vi "Tone (G3)-Create.vi"(0 "Tone Class in":T1, 5 "Sampling Rate (Hz)":dbl, 7 "Npts":i32, 9 "RepNum":i32, 11 "error in (no error)":errorcluster) -> (4 "Tone Class out":T1, 6 "Waveform":dbl[](array[numeric]), 15 "error out":errorcluster)   [LabVIEW 2020]
uses:
  Tone.Properties.ctl
  <vilib>/Analysis/NI_AALBase.lvlib
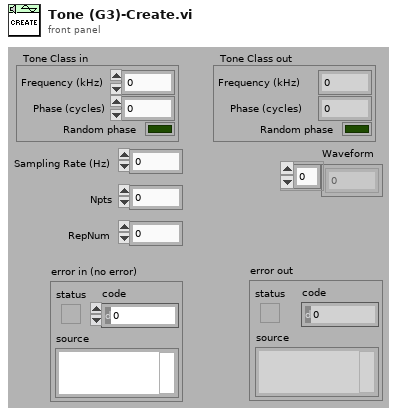
[diagram p1: front panel]
types:
  T1 = typedef "Tone.Properties.ctl" = cluster{"Frequency (kHz)":dbl, "Phase (cycles)":dbl, "Random phase":bool}
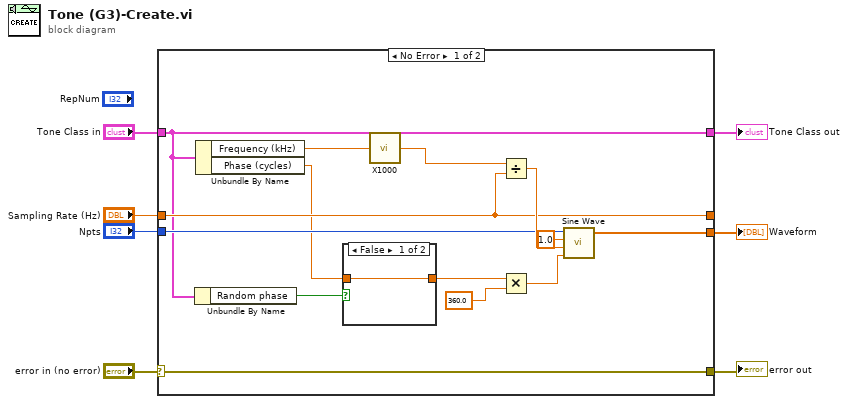
[diagram p0: block diagram]
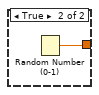
[diagram p2: hidden frame]
diagram:
  n1 = case shown="No Error" "error in (no error)" {
    selector: "error in (no error)" -> [w21 w26]
    tunnel: [w21 w26] -> w6
    tunnel: [w12 w25] -> w4
    tunnel: "Tone Class in" -> [w12 w25]
    tunnel: "Npts" -> [w16 _]
    tunnel: "Sampling Rate (Hz)" -> [w17 w24]
    tunnel: [w18 _] -> w1
    tunnel: [w17 w24] -> _
    frame No Error {
      n2 = Unbundle By Name(w12) -> ("Random phase"=w11:bool)
      n3 = Unbundle By Name(w12) -> ("Frequency (kHz)"=w14:dbl, "Phase (cycles)"=w10:dbl)
      n4 = case shown="False" w11 {
        tunnel: w10 -> [w22 _]
        tunnel: [w22 w23] -> w9
        frame False {
        }
        frame True {
          n5 = Random Number (0-1)() -> (number: 0 to 1=w23:dbl)
        }
      }
      n6 = call "X1000.vi"("X"=w14) -> ("X/1000"=w15:dbl)
      n7 = Divide(x=w15, y=w17) -> (x/y=w19:dbl)
      n8 = Multiply(x=w9, y=360.0) -> (x*y=w8:dbl)
      n9 = call <vilib>:"Sine Wave.vi"("samples"=w16, "amplitude"=1.0, "frequency"=w19, "phase in"=w8) -> ("sine wave"=w18:dbl[])  [unwired: 1 in, 2 out]
    }
    frame Error {
    }
  }
  "error out" <- w6
  "Tone Class out" <- w4
  "Waveform" <- w1
